vi "Edit Data Interactively.vi"(8 "error in (no error)":errorcluster, 11 "Data Item in":refnum<class "Data Item.lvclass">) -> (0 "error out":errorcluster, 3 "Data Item out":refnum<class "Data Item.lvclass">)   [LabVIEW 2018, in "VILab.lvlib" / "Data Item.lvclass"]
uses:
  Data Item.lvclass
  Data Item.lvclass/Data Item.ctl
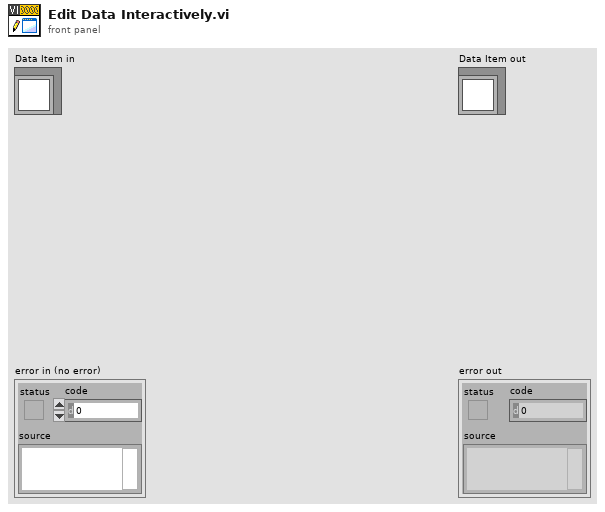
[diagram p1: front panel]
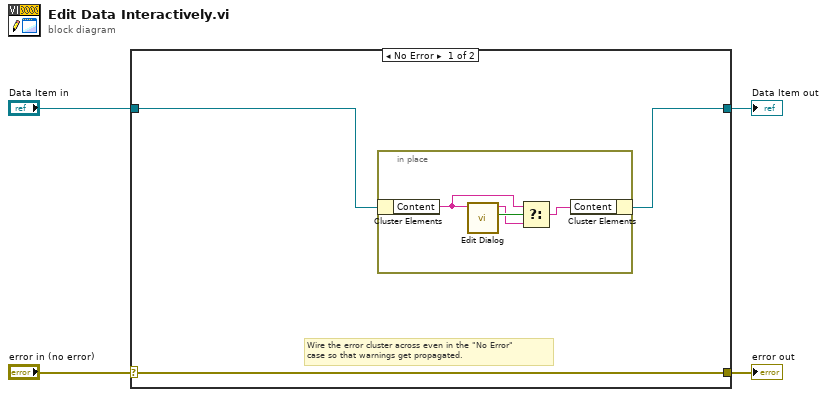
[diagram p0: block diagram]
diagram:
  n1 = case shown="No Error" "error in (no error)" {
    selector: "error in (no error)" -> [w7 w13]
    tunnel: [w7 w13] -> w3
    tunnel: [w5 w12] -> w1
    tunnel: "Data Item in" -> [w6 w12]
    frame No Error {
      # "Wire the error cluster across even in the \"No Error\"\ncase so that warnings get propagated."
      n2 = in-place {
        n3 = in-place-cluster #1(w6) -> ("Content"=w8:string)
        n4 = call "Edit Dialog.vi"("Content"=w8) -> ("Canceled?"=w11:bool, "String"=w10:string)  [unwired: 9 in]
        n5 = Select(t=w8, s=w11, f=w10) -> (s? t:f=w9:string)
        n6 = in-place-cluster #1("Content"=w9) -> (w5:refnum<class "Data Item.lvclass">)
      }
    }
    frame Error {
    }
  }
  "error out" <- w3
  "Data Item out" <- w1
